vi "Week1_Exercise2.vi"() -> ()   [LabVIEW 2015]
panel:
  in  "stop":bool
  out "s? t:f":string
  in  "Person B":dbl
  in  "Person A":dbl
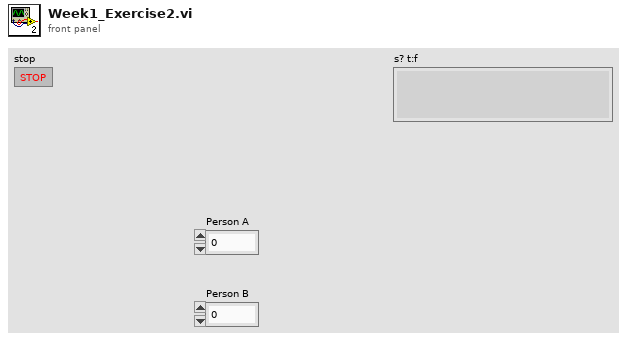
[diagram p1: front panel]
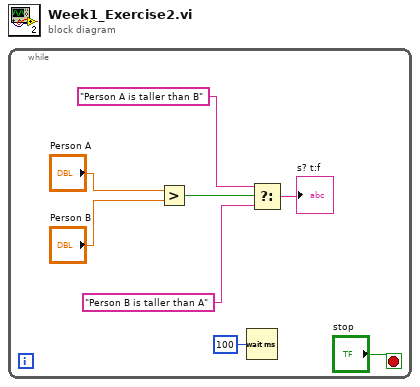
[diagram p0: block diagram]
diagram:
  n1 = while {
    stop <- "stop" stop-if-true
    n2 = Greater?(x="Person A", y="Person B") -> (0:w6:bool)
    n3 = Wait (ms)(milliseconds to wait=u32 100) -> ()  [unwired: 1 out]
    n4 = Select(t="Person A is taller than B", s=w6, f="Person B is taller than A") -> (s? t:f=→"s? t:f":string)
  }
